vi "10.3 Writing multichannel Data to a file.vi"() -> ()   [LabVIEW 2019]
uses:
  <vilib>/DAQmx/read.llb/DAQmx Read (Analog 1D DBL NChan 1Samp).vi
  <vilib>/DAQmx/create/channels.llb/DAQmx Create Channel (AI-Temperature-Thermocouple).vi
  <vilib>/DAQmx/configure/timing.llb/DAQmx Timing (Sample Clock).vi
  <vilib>/DAQmx/miscellaneous.llb/DAQmx Fill In Error Info.vi
panel:
  in  "Configuration Control":T1={"number of samples"=-1, "Minimum Value"=-1.0, "Maximum Value"=-1.0, "physical channels"="Multi_I-O/ai0", "Desired Sample Rate (Hz)"=-1.0, "sample mode"=10178} {"sample mode" items=["Finite Samples"=10178, "Continuous Samples"=10123, "Hardware Timed Single Point"=12522]}
  in  "File Path Control":path
  in  "Stop":bool
  out "Waveform Chart":T2(graph)
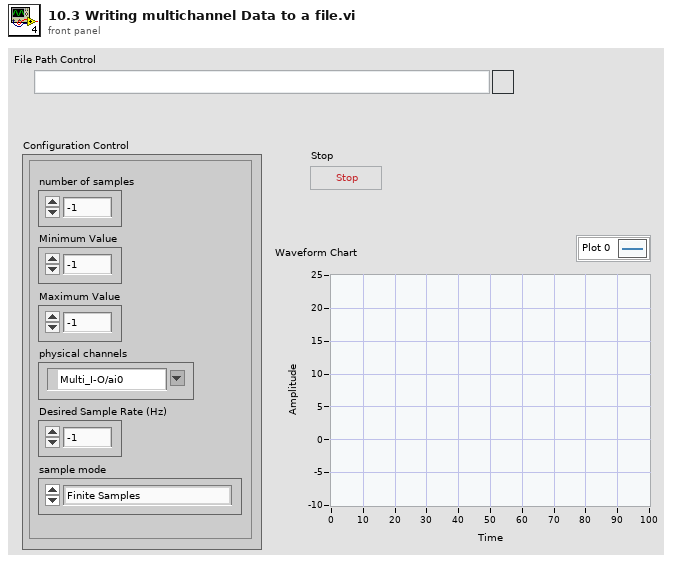
[diagram p1: front panel]
types:
  T1 = cluster{"number of samples":i32, "Minimum Value":dbl, "Maximum Value":dbl, "physical channels":tag, "Desired Sample Rate (Hz)":dbl, "sample mode":i32}
  T2 = cluster{"data[0]":dbl, "data[1]":dbl, "data[2]":dbl, "data[3]":dbl, "data[4]":dbl, "data[5]":dbl, "data[6]":dbl, "data[7]":dbl, "data[8]":dbl}
  T3 = enum16{"open", "replace", "create", "open or create", "replace or create", "replace or create with confirmation"}
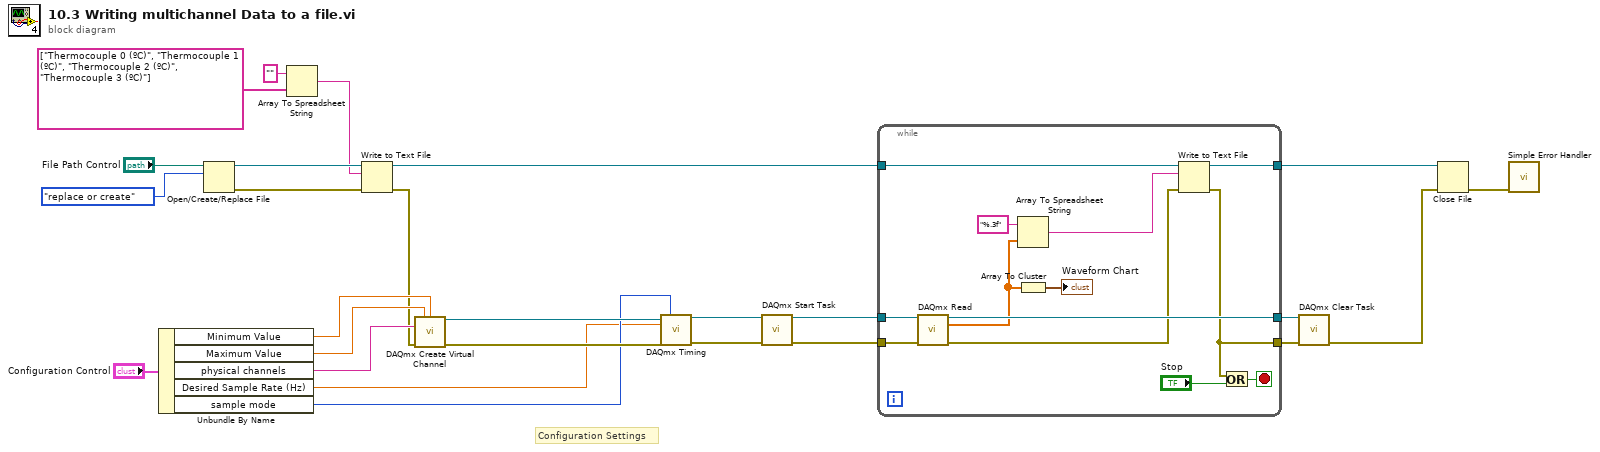
[diagram p0: block diagram]
diagram:
  # "Configuration Settings"
  n1 = Unbundle By Name("Configuration Control") -> ("Minimum Value"=w9:dbl, "Maximum Value"=w10:dbl, "physical channels"=w8:tag, "Desired Sample Rate (Hz)"=w6:dbl, "sample mode"=w7:i32)
  n2 = Open/Create/Replace File(file path (use dialog)="File Path Control", operation (0:open)=T3."replace or create") -> (refnum out=w20:refnum<file>, error out=w19:errorcluster)  [unwired: 4 in, 1 out]
  n3 = Array To Spreadsheet String(array=string[] ["Thermocouple 0 (ºC)", "Thermocouple 1 (ºC)", "Thermocouple 2 (ºC)", "Thermocouple 3 (ºC)"], 3:"" ("format string")) -> (spreadsheet string=w18:string)  [unwired: 1 in]
  n4 = Write to Text File(file (use dialog)=w20, text=w18, error in=w19) -> (refnum out=w17:refnum<file>, error out=w4:errorcluster)  [unwired: 1 in, 1 out]
  n5 = call-poly <vilib>:"DAQmx Create Virtual Channel.vi"("maximum value"=w10, "minimum value"=w9, "physical channels"=w8, "error in"=w4) -> ("task out"=w13:refnum<k21>, "error out"=w12:errorcluster)  [unwired: 10 in]
  n6 = call-poly <vilib>:"DAQmx Timing.vi"("task/channels in"=w13, "sample mode"=w7, "rate"=w6, "error in"=w12) -> ("task out"=w3:refnum<k21>, "error out"=w5:errorcluster)  [unwired: 10 in]
  n7 = call <vilib>:"DAQmx Start Task.vi"("task/channels in"=w3, "error in"=w5) -> ("task out"=w26:refnum<k21>, "error out"=w24:errorcluster)  [unwired: 12 in]
  n8 = while {
    tunnel: w26 -> [w39]
    tunnel: [w38] -> w25
    tunnel: w24 -> [w37]
    tunnel: [w33] -> w23
    tunnel: w17 -> [w34]
    tunnel: [w32] -> w16
    stop <- w36 stop-if-true
    n9 = call-poly <vilib>:"DAQmx Read.vi"("task/channels in"=w39, "error in"=w37) -> ("task out"=w38:refnum<k21>, "data"=w31:dbl[], "error out"=w28:errorcluster)  [unwired: 11 in]
    n10 = Array To Spreadsheet String(array=w31, 3:"%.3f" ("format string")) -> (spreadsheet string=w27:string)  [unwired: 1 in]
    n11 = Array To Cluster(array=w31) -> (cluster=→"Waveform Chart":T2)
    n12 = Write to Text File(file (use dialog)=w34, text=w27, error in=w28) -> (refnum out=w32:refnum<file>, error out=w33:errorcluster)  [unwired: 1 in, 1 out]
    n13 = Or(x=w33, y="Stop") -> (x .or. y?=w36:bool)
  }
  n14 = call <vilib>:"DAQmx Clear Task.vi"("task in"=w25, "error in"=w23) -> ("error out"=w15:errorcluster)  [unwired: 13 in]
  n15 = Close File(refnum=w16, error in=w15) -> (error out=w14:errorcluster)  [unwired: 1 out]
  n16 = call <vilib>:"Simple Error Handler.vi"("error in (no error)"=w14) -> ()  [unwired: 4 in, 5 out]
